vi "Set All Channels.vi"(8 "error in (no error)":errorcluster, 10 "Channels in":T1[](array[typedef]), 11 "VISA Refnum in":refnum<visa-resource-name>="COM1") -> (0 "error out":errorcluster, 2 "Channels out":T1[](array[typedef]), 3 "VISA Refnum out":refnum<visa-resource-name>)   [LabVIEW 2019, in "KH7008.lvlib"]
uses:
  KH7008.lvlib
  typedefs/SetAll--Cluster.ctl
  typedefs/Channel--Enum.ctl
  typedefs/Gain--Enum.ctl
  typedefs/Input Configuration--Enum.ctl
  typedefs/Shunt--Enum.ctl
  typedefs/Coupling--Enum.ctl
  typedefs/Filter--Enum.ctl
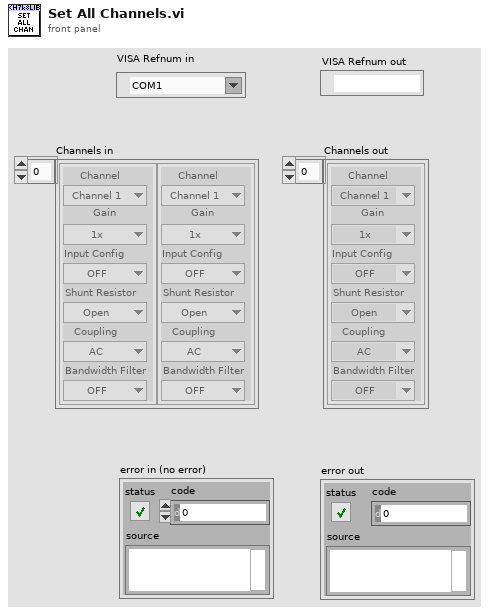
[diagram p1: front panel]
types:
  T1 = typedef "KH7008.lvlib/SetAll--Cluster.ctl" = cluster{"Channel":T2, "Gain":T3, "Input Config":T4, "Shunt Resistor":T5, "Coupling":T6, "Bandwidth Filter":T7}
  T2 = typedef "KH7008.lvlib/Channel--Enum.ctl" = enum8{"Channel 1", "Channel 2", "Channel 3", "Channel 4", "Channel 5", "Channel 6", "Channel 7", "Channel 8"}
  T3 = typedef "KH7008.lvlib/Gain--Enum.ctl" = enum8{"1x", "10x", "100x", "1000x"}
  T4 = typedef "KH7008.lvlib/Input Configuration--Enum.ctl" = enum8{"OFF", "SE+", "SE-", "DIFF"}
  T5 = typedef "KH7008.lvlib/Shunt--Enum.ctl" = enum8{"Open", "50 Ohms", "500 Ohms", "5k Ohms", "50k Ohms", "10M Ohm"}
  T6 = typedef "KH7008.lvlib/Coupling--Enum.ctl" = enum8{"AC", "DC"}
  T7 = typedef "KH7008.lvlib/Filter--Enum.ctl" = enum8{"OFF", "ON"}
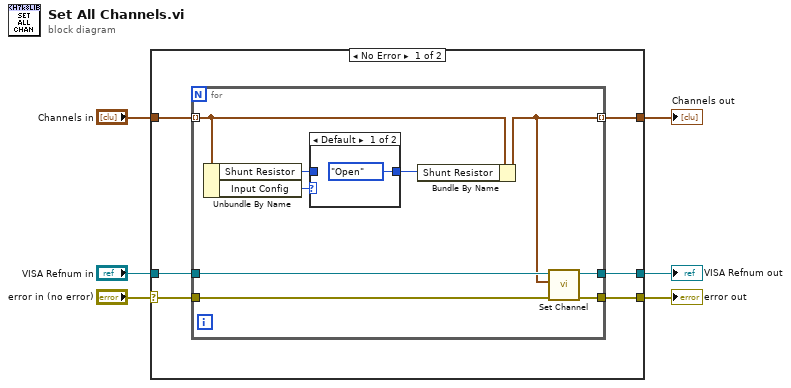
[diagram p0: block diagram]
diagram:
  n1 = case shown="No Error" "error in (no error)" {
    selector: "error in (no error)" -> [w9 w26]
    tunnel: "Channels in" -> [w12 w24]
    tunnel: "VISA Refnum in" -> [w11 w25]
    tunnel: [w10 w26] -> w4
    tunnel: [w8 w25] -> w2
    tunnel: [w7 w24] -> w1
    frame No Error {
      n2 = for {
        tunnel: w12 -> [w15] mode=indexing
        tunnel: [w13] -> w7 mode=indexing
        tunnel: w11 -> [w20]
        tunnel: [w14] -> w8
        tunnel: w9 -> [w17]
        tunnel: [w21] -> w10
        n3 = Unbundle By Name(w15) -> ("Shunt Resistor"=w19:T5, "Input Config"=w18:T4)
        n4 = case shown="Default" w18 {
          tunnel: [Shunt--Enum."Open" ("f") w23] -> w16
          tunnel: w19 -> [_ w23]
          frame Default {
          }
          frame "DIFF" {
          }
        }
        n5 = Bundle By Name(cluster=w15, "Shunt Resistor"=w16) -> (w13:T1)
        n6 = call "Set Channel.vi"("error in (no error)"=w17, "Channel Parameters"=w13, "VISA Refnum in"=w20) -> ("error out"=w21:errorcluster, "VISA Refnum out"=w14:refnum<visa-resource-name>)  [unwired: 7 in]
      }
    }
    frame Error {
    }
  }
  "error out" <- w4
  "VISA Refnum out" <- w2
  "Channels out" <- w1
